vi "Servos (Alice).vi"(10 "Servo 2:":dbl, 11 "Servo 1:":dbl) -> ()   [LabVIEW 2013]
uses:
  <vilib>/LabVIEW Interface for Arduino/LabVIEW Interface for Arduino.lvlib
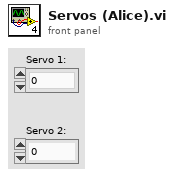
[diagram p1: front panel]
types:
  T1 = typedef "LabVIEW Interface for Arduino.lvlib/Arduino Resource.ctl" = cluster{"VISA resource":refnum<visa-resource-name>, "Board Type":T2, "Connection Type":enum8{"USB / Serial"}, "Bytes Per Packet (15)":u8}
  T2 = typedef "LabVIEW Interface for Arduino.lvlib/Board Type.ctl" = enum16{"Uno", "Dimuelanove w/Atmega 328", "Mega 2560"}
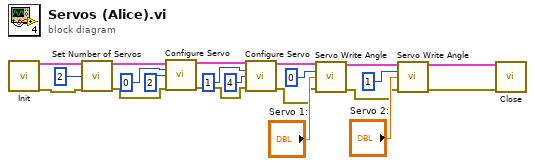
[diagram p0: block diagram]
diagram:
  n1 = call <vilib>:"Init.vi"() -> ("Arduino Resource"=w21:T1, "error out"=w13:errorcluster)  [unwired: 18 in]
  n2 = call <vilib>:"Set Number of Servos.vi"("Arduino Resource"=w21, "Number Of Servos (1)"=2, "error in"=w13) -> ("Arduino Resource"=w9:T1, "error out"=w3:errorcluster)  [unwired: 11 in]
  n3 = call <vilib>:"Configure Servo.vi"("Arduino Resource"=w9, "Servo Number (0)"=0, "DIO Pin (2)"=2, "error in"=w3) -> ("Arduino Resource"=w7:T1, "error out"=w2:errorcluster)  [unwired: 10 in]
  n4 = call <vilib>:"Configure Servo.vi"("Arduino Resource"=w7, "Servo Number (0)"=1, "DIO Pin (2)"=4, "error in"=w2) -> ("Arduino Resource"=w6:T1, "error out"=w1:errorcluster)  [unwired: 10 in]
  n5 = call <vilib>:"Servo Write Angle.vi"("Arduino Resource"=w6, "Servo Number"=0, "Angle (Degrees)"="Servo 1:", "error in"=w1) -> ("Arduino Resource"=w17:T1, "error out"=w12:errorcluster)  [unwired: 10 in]
  n6 = call <vilib>:"Servo Write Angle.vi"("Arduino Resource"=w17, "Servo Number"=1, "Angle (Degrees)"="Servo 2:", "error in"=w12) -> ("Arduino Resource"=w14:T1, "error out"=w11:errorcluster)  [unwired: 10 in]
  n7 = call <vilib>:"Close.vi"("Arduino Resource"=w14, "error in"=w11) -> ()  [unwired: 13 in, 1 out]
